vi "异常处理作业.vi"() -> ()   [LabVIEW 2023]
panel:
  out "Waveform Graph":dynamicdata(graph)
  out "error out":errorcluster
  in  "Numeric":dbl
  # "异常处理 作业"
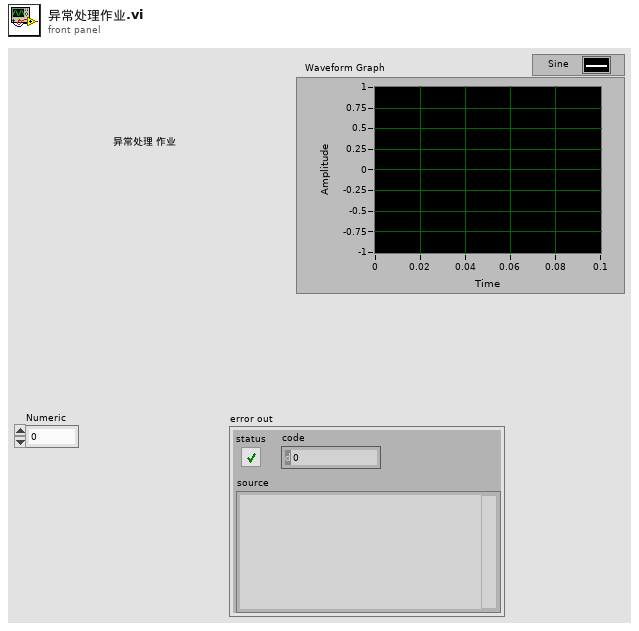
[diagram p1: front panel]
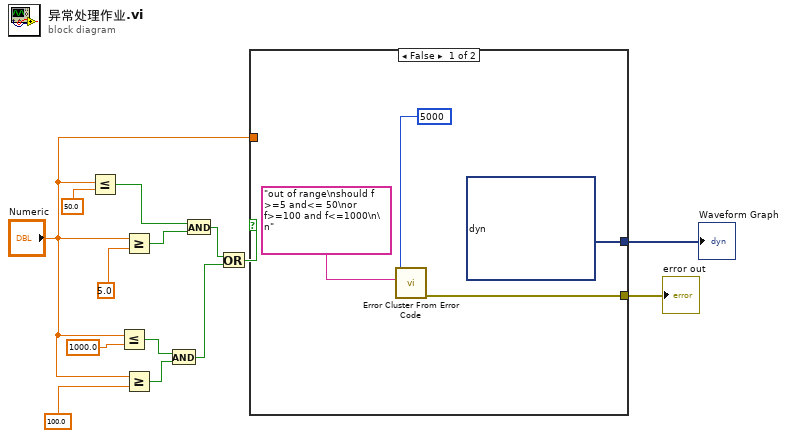
[diagram p0: block diagram]
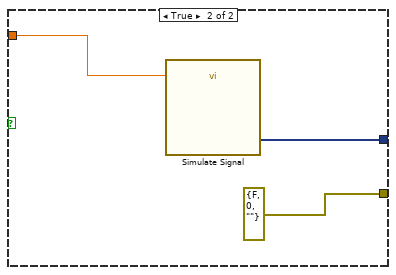
[diagram p2: hidden frame]
diagram:
  n1 = Less Or Equal?(x="Numeric", y=50.0) -> (x <= y?=w12:bool)
  n2 = Less Or Equal?(x="Numeric", y=1000.0) -> (x <= y?=w5:bool)
  n3 = Greater Or Equal?(x="Numeric", y=5.0) -> (x >= y?=w11:bool)
  n4 = Greater Or Equal?(x="Numeric", y=100.0) -> (x >= y?=w4:bool)
  n5 = And(x=w5, y=w4) -> (x .and. y?=w2:bool)
  n6 = And(x=w12, y=w11) -> (x .and. y?=w3:bool)
  n7 = Or(x=w3, y=w2) -> (x .or. y?=w1:bool)
  n8 = case shown="False" w1 {
    tunnel: "Numeric" -> [_ w21]
    tunnel: [w16 errorcluster {"status"=FALSE, "code"=0, "source"=""} ("error constant")] -> w10
    tunnel: [dynamicdata [] ("Sine") w19] -> w9
    frame False {
      n9 = call <vilib>:"Error Cluster From Error Code.vi"("error message (\"\")"="out of range\nshould f >=5 and<= 50\nor f>=100 and f<=1000\n\n" ("error message (\"\")"), "error code (0)"=5000) -> ("error out"=w16:errorcluster)  [unwired: 7 in]
    }
    frame True {
      n10 = call "Simulate Signal"("Frequency"=w21) -> ("Sine"=w19:dynamicdata)  [unwired: 13 in, 1 out]
    }
  }
  "error out" <- w10
  "Waveform Graph" <- w9
